vi "Report Tool2.vi"(0 "name or relative path":string=".csv", 1 "Files":path[](array[path]), 5 "base path":path=path "C:/RageATE Results", 13 "WriteToFile(t)":bool=TRUE) -> (4 "reportfile(str)":string="C:\\RageATE Results\\1234.csv.csv")   [LabVIEW 2018]
uses:
  <vilib>/Utility/file.llb/Read Delimited Spreadsheet (string).vi
  <vilib>/Utility/file.llb/Write Delimited Spreadsheet (string).vi
panel:
  out "file or folder exists?":bool
  out "reportfile":path=path "C:/RageATE Results/1234.csv.csv"
  out "Tx-Att_Test Name":string
  out "Tx_Test Name":string
  in  "RunRx(t)":bool=TRUE
  in  "RunTx(t)":bool=TRUE
  in  "RunATTEN(t)":bool=TRUE
  in  "error in (no error)":errorcluster
  out "error out":errorcluster
  out "TX-ATT_DAT":string[][](array[string])=[["#Test Name:", "REV-C_TETRA_TX-ATTEN"], ["#MSN:", "RGE2100000"], ["#ESN:", "xxxxxxxx"], ["#TestOperator:", "411 WATSON T NBPT"], ["#Test_Bench_Name:", "WAM_PROD_TEST-1"], ["#Test Parameters File Name:", "'C:\\RageATE\\Automated Tests\\Tetra WAM\\PRODUCTION\\setup files\\WAM-C_TX-ATTEN_Parameters.tst'"], ["#Gitlog Commit:", "41159ffc8fe9c2318ec8f6db4e89b94d30bdf9e8"], ["#LotID:", "2228"], ["#SW_Version:", "02000005"], ["#Result File Path:", "'C:\\RageATE Results\\REV-C_TETRA_TX-ATTEN\\7_11_2022\\REV-C_TETRA_TX-ATTEN_SN_RGE2100000_ 2228_071122-130320.csv'"], ["%TX_ATT", "PASS"]]
  out "TX_ATT":string="PASS"
  out "TxAtt_DataLength":i32=24
  out "TxAtt_Result":i32[][](array[numeric])=[[1], [1], [1], [1], [1], [1], [1], [1], [1], [1], [1], [1], [1], [1], [1], [1], [1], [1], [1], [1], [1], [1], [1], [1]]
  out "TxAtt_DataHeaderRow":i32=45
  out "TxAtt_Header_data":string[](array[string])=["REV-C_TETRA_TX-ATTEN", "RGE2100000", "xxxxxxxx", "411 WATSON T NBPT", "WAM_PROD_TEST-1", "'C:\\RageATE\\Automated Tests\\Tetra WAM\\PRODUCTION\\setup files\\WAM-C_TX-ATTEN_Parameters.tst'", "41159ffc8fe9c2318ec8f6db4e89b94d30bdf9e8", "2228", "02000005", "'C:\\RageATE Results\\REV-C_TETRA_TX-ATTEN\\7_11_2022\\REV-C_TETRA_TX-ATTEN_SN_RGE2100000_ 2228_071122-130320.csv'"]
  out "TxAtt_Header":string[](array[string])=["#Test Name:", "#MSN:", "#ESN:", "#TestOperator:", "#Test_Bench_Name:", "#Test Parameters File Name:", "#Gitlog Commit:", "#LotID:", "#SW_Version:", "#Result File Path:"]
  out "TXAtt_ResultFile":string="C:\\RageATE Results\\REV-C_TETRA_TX-ATTEN\\7_11_2022\\REV-C_TETRA_TX-ATTEN_SN_RGE2100000_ 2228_071122-130320.csv"
  in  "TX_PROD_ATTEN":path=path "C:/RageATE Results/REV-C_TETRA_TX-ATTEN/7_11_2022/REV-C_TETRA_TX-ATTEN_SN_RGE2100000_ 2228_071122-130320.csv"
  out "TxAtt_Data":string[][](array[string])
  out "TX_FLAT":string="FAIL *12"
  out "RX_DAT":string[][](array[string])=[["#Test Name:", "REV-C_TETRA_RX-PROD"], ["#MSN:", "RGE2100000"], ["#ESN:", "xxxxxxxx"], ["#TestOperator:", "411 WATSON T NBPT"], ["#Test_Bench_Name:", "WAM_PROD_TEST-1"], ["#Test Parameters File Name:", "'C:\\RageATE\\Automated Tests\\Tetra WAM\\PRODUCTION\\setup files\\WAM-C_RX-PROD_Parameters.tst'"], ["#Gitlog Commit:", "41159ffc8fe9c2318ec8f6db4e89b94d30bdf9e8"], ["#LotID:", "2228"], ["#SW_Version: ", "02000005"], ["#Result File Path:", "'C:\\RageATE Results\\REV-C_TETRA_RX-PROD\\7_11_2022\\REV-C_TETRA_RX-PROD_SN_RGE2100000_ 2228_071122-132555.csv'"], ["%RX_DC", "PASS"], ["%RX_GAIN", "PASS"], ["%RX_NF", "FAIL *34"]]
  out "RX_DC":string="PASS"
  out "RX_G":string="PASS"
  out "RX_NF":string="FAIL *34"
  out "Rx_DataLength":i32=1608
  out "Rx_Result":i32[][](array[numeric])
  out "Rx_DataHeaderRow":i32=45
  out "Rx_Header_data":string[](array[string])=["REV-C_TETRA_RX-PROD", "RGE2100000", "xxxxxxxx", "411 WATSON T NBPT", "WAM_PROD_TEST-1", "'C:\\RageATE\\Automated Tests\\Tetra WAM\\PRODUCTION\\setup files\\WAM-C_RX-PROD_Parameters.tst'", "41159ffc8fe9c2318ec8f6db4e89b94d30bdf9e8", "2228", "02000005", "'C:\\RageATE Results\\REV-C_TETRA_RX-PROD\\7_11_2022\\REV-C_TETRA_RX-PROD_SN_RGE2100000_ 2228_071122-132555.csv'"]
  out "Rx_Header":string[](array[string])=["#Test Name:", "#MSN:", "#ESN:", "#TestOperator:", "#Test_Bench_Name:", "#Test Parameters File Name:", "#Gitlog Commit:", "#LotID:", "#SW_Version: ", "#Result File Path:"]
  out "RX_ResultFile":string="C:\\RageATE Results\\REV-C_TETRA_RX-PROD\\7_11_2022\\REV-C_TETRA_RX-PROD_SN_RGE2100000_ 2228_071122-132555.csv"
  in  "RX_PROD_FILE":path=path "C:/RageATE Results/REV-C_TETRA_RX-PROD/7_11_2022/REV-C_TETRA_RX-PROD_SN_RGE2100000_ 2228_071122-132555.csv"
  out "Rx_Data":string[][](array[string])
  out "Tx_Result":i32[][](array[numeric])
  out "Tx_DataLength":i32=2412
  out "Tx_Header":string[](array[string])=["#Test Name:", "#ESN:", "#MSN:", "#TestOperator:", "#Test_Bench_Name:", "#Test Parameters File Name:", "#Gitlog Commit:", "#LotID:", "#SW_Version: ", "#Result File Path:"]
  out "Tx_Data":string[][](array[string])
  out "TX_DAT":string[][](array[string])=[["#Test Name:", "REV-C_TETRA_TX-PROD"], ["#ESN:", "xxxxxxxx"], ["#MSN:", "RGE2100000"], ["#TestOperator:", "411 WATSON T NBPT"], ["#Test_Bench_Name:", "WAM_PROD_TEST-1"], ["#Test Parameters File Name:", "'C:\\RageATE\\Automated Tests\\Tetra WAM\\PRODUCTION\\setup files\\WAM-C_TX-PROD_Parameters.tst'"], ["#Gitlog Commit:", "41159ffc8fe9c2318ec8f6db4e89b94d30bdf9e8"], ["#LotID:", "2228"], ["#SW_Version: ", "02000005"], ["#Result File Path:", "'C:\\RageATE Results\\REV-C_TETRA_TX-PROD\\7_11_2022\\REV-C_TETRA_TX-PROD_SN_RGE2100000_ 2228_071122-130423.csv'"], ["%TX_DC", "PASS"], ["%TX_POW", "FAIL *1301"], ["%TX_S11", "FAIL *125"], ["%TX_H2", "PASS"], ["%TX_FLAT", "FAIL *12"]]
  out "Tx_Header_data":string[](array[string])=["REV-C_TETRA_TX-PROD", "xxxxxxxx", "RGE2100000", "411 WATSON T NBPT", "WAM_PROD_TEST-1", "'C:\\RageATE\\Automated Tests\\Tetra WAM\\PRODUCTION\\setup files\\WAM-C_TX-PROD_Parameters.tst'", "41159ffc8fe9c2318ec8f6db4e89b94d30bdf9e8", "2228", "02000005", "'C:\\RageATE Results\\REV-C_TETRA_TX-PROD\\7_11_2022\\REV-C_TETRA_TX-PROD_SN_RGE2100000_ 2228_071122-130423.csv'"]
  in  "TX_PROD_FILE":path=path "C:/RageATE Results/REV-C_TETRA_TX-PROD/7_11_2022/REV-C_TETRA_TX-PROD_SN_RGE2100000_ 2228_071122-130423.csv"
  out "TX_ResultFile":string="C:\\RageATE Results\\REV-C_TETRA_TX-PROD\\7_11_2022\\REV-C_TETRA_TX-PROD_SN_RGE2100000_ 2228_071122-130423.csv"
  out "Tx_DataHeaderRow":i32=45
  out "Rx_Test Name":string
  out "TX_H2":string="PASS"
  out "TX_S11":string="FAIL *125"
  out "TX_POW":string="FAIL *1301"
  out "TX_DC":string="PASS"
  # "C:\\RageATE Results\\REV-C_TETRA_TX-ATTEN\\7_11_2022\\REV-C_TETRA_TX-ATTEN_SN_RGE2100000_ 2228_071122-130320.csv"
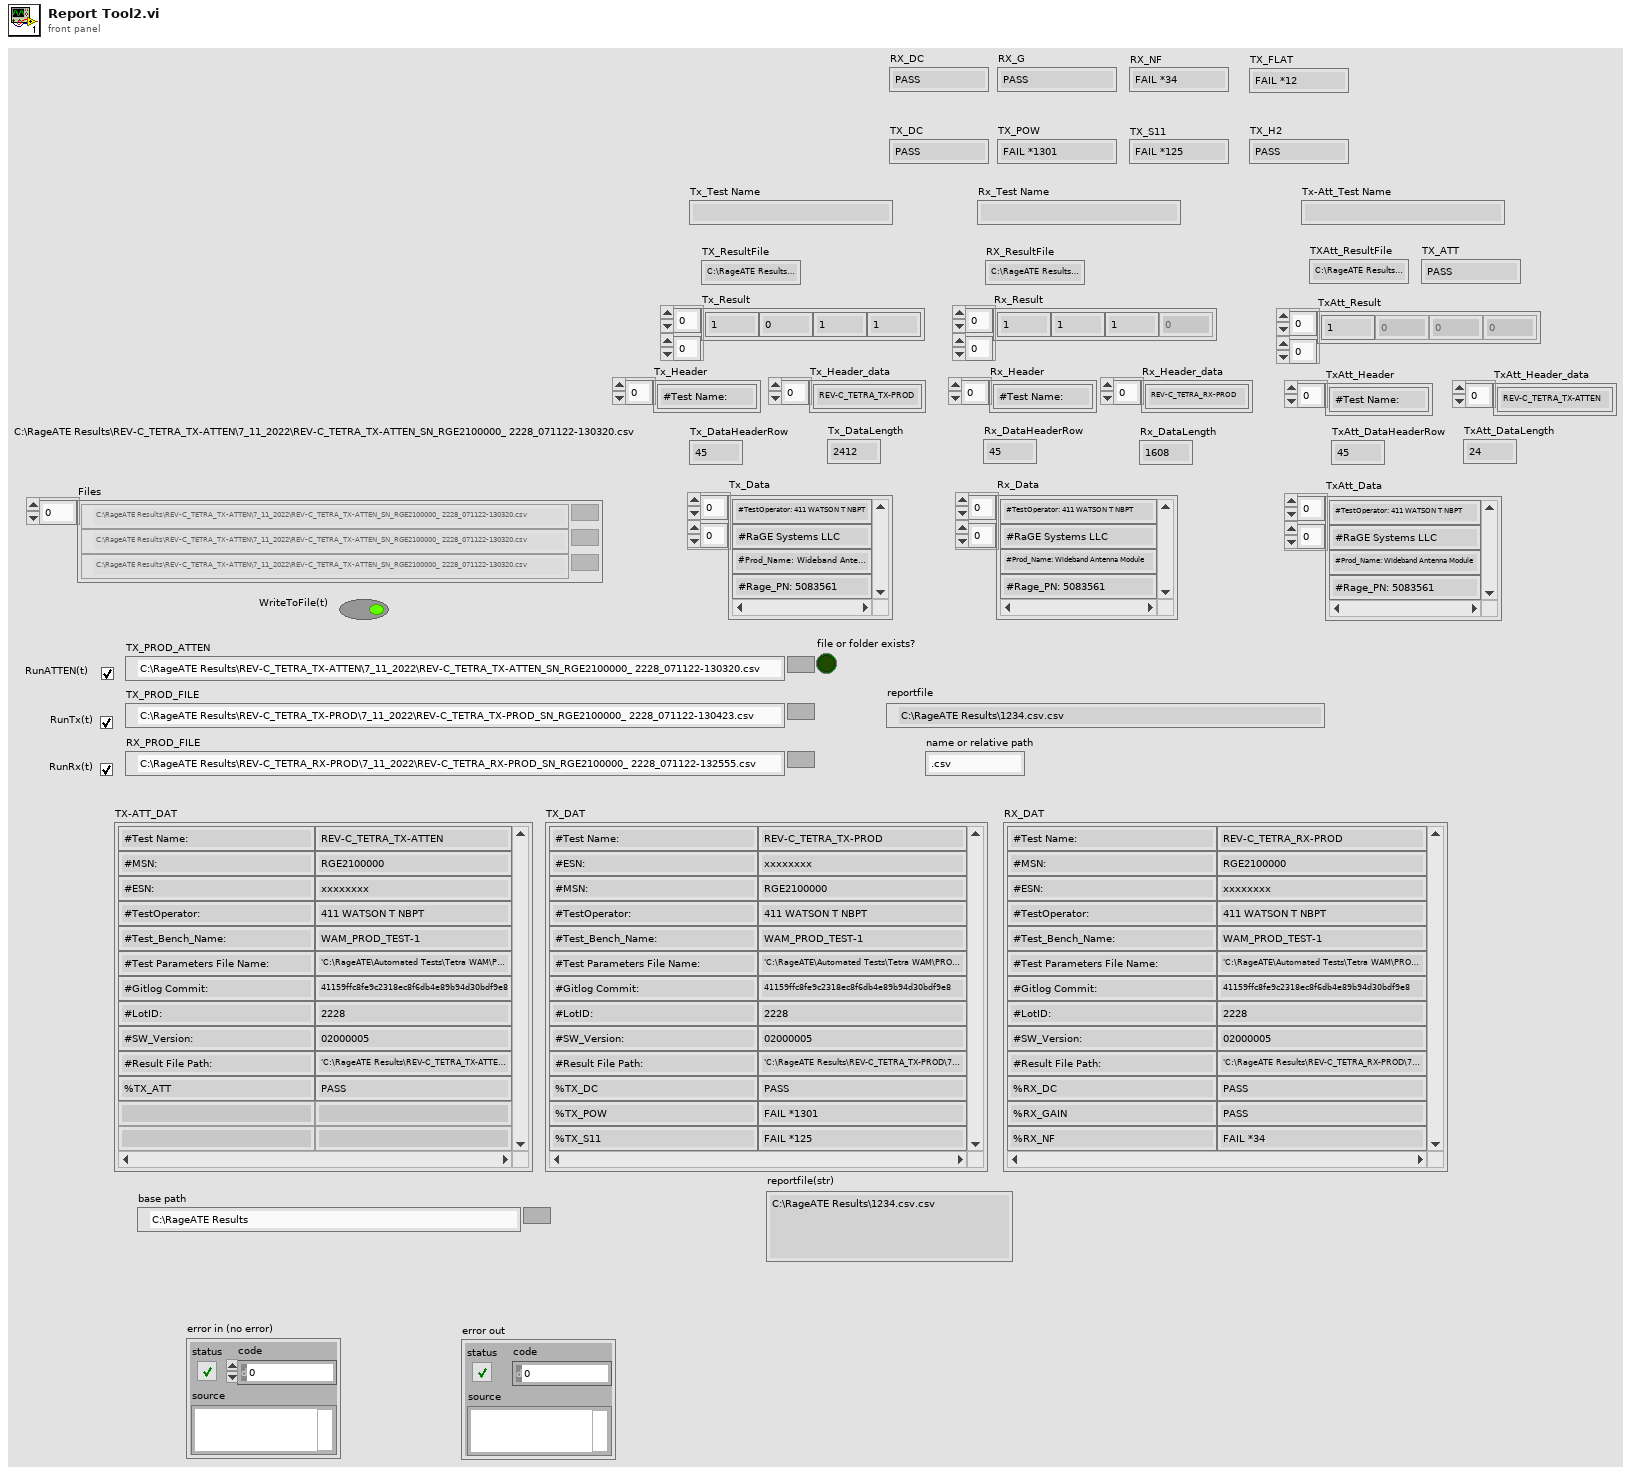
[diagram p1: front panel]
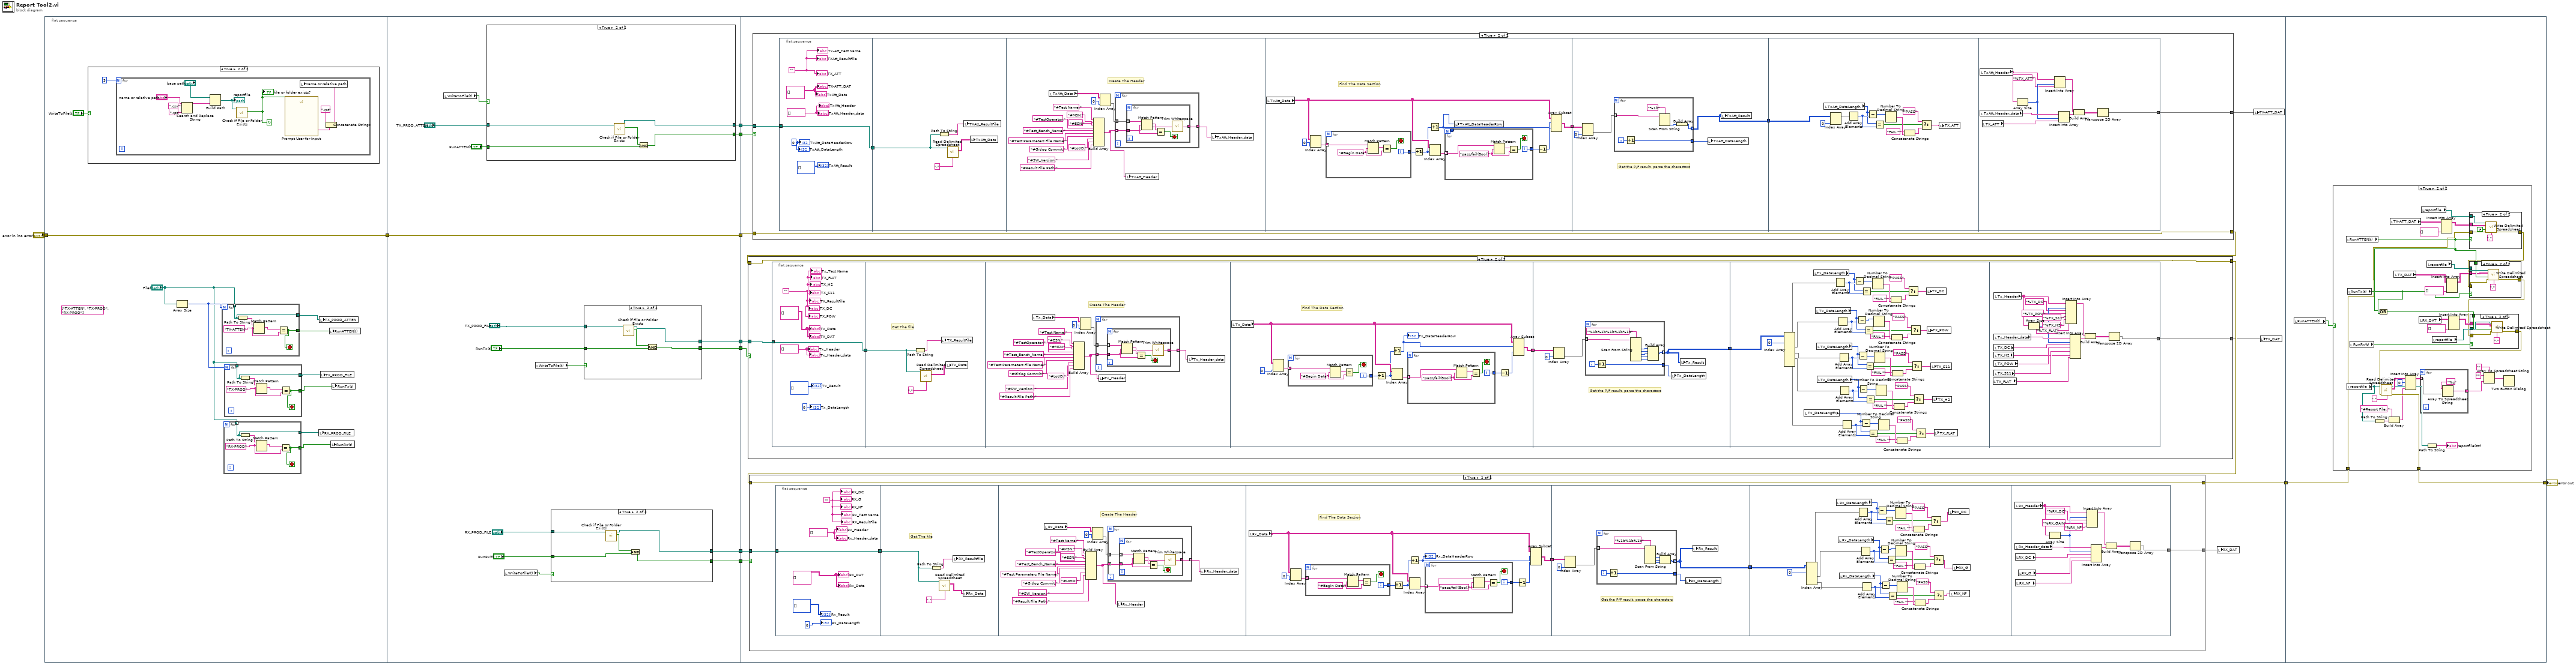
[diagram p0: block diagram]
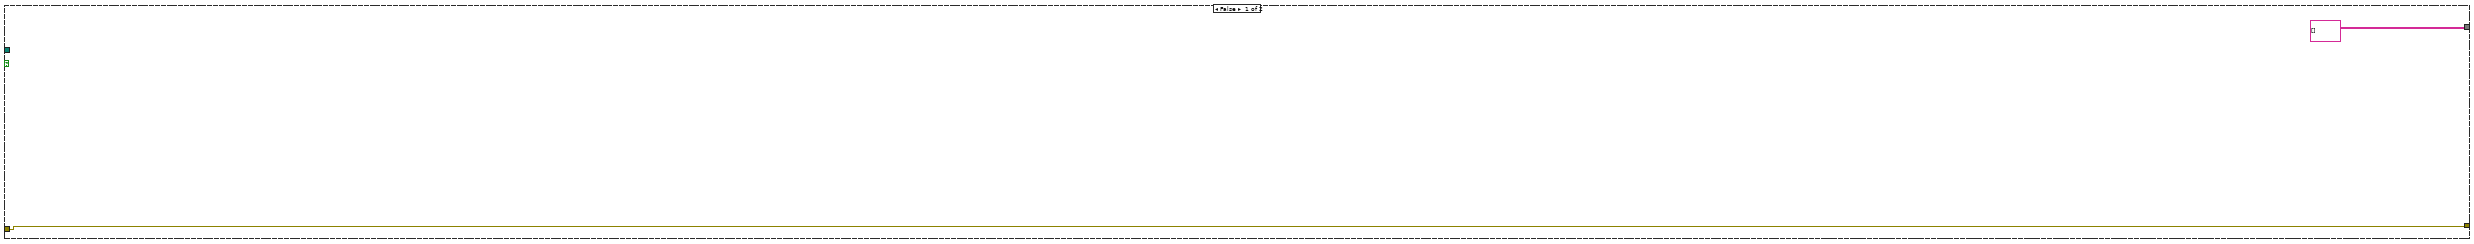
[diagram p6: hidden frame]
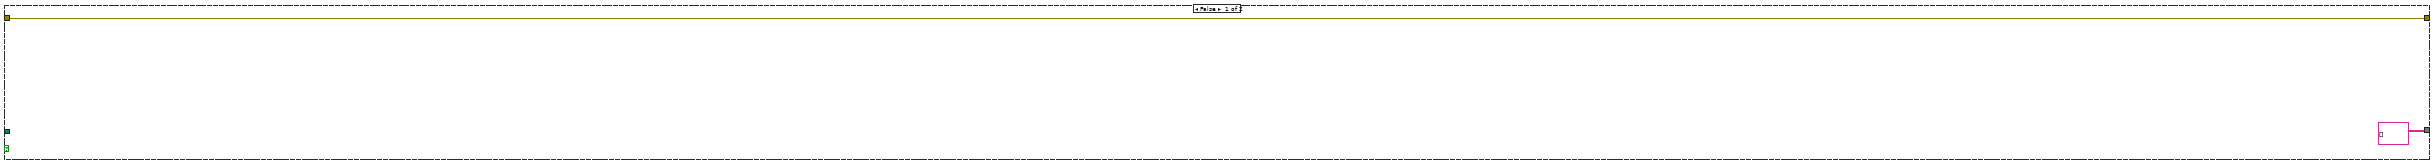
[diagram p7: hidden frame]
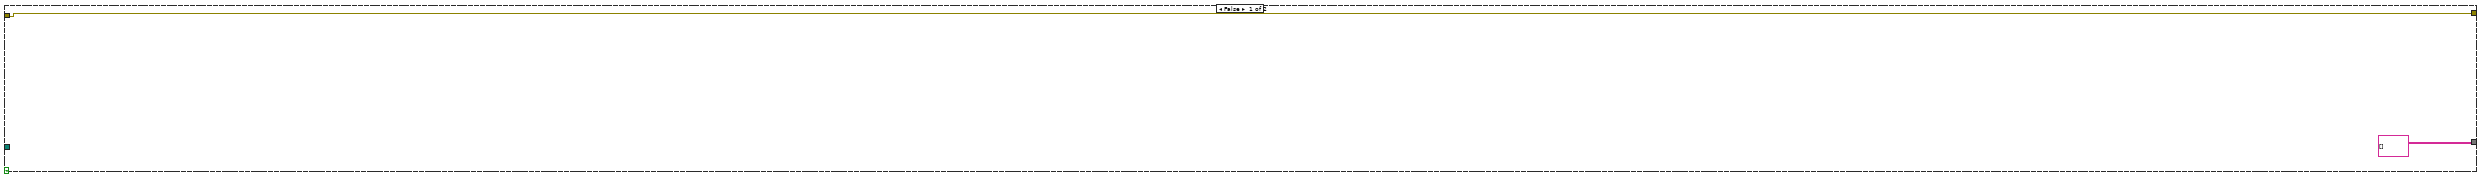
[diagram p8: hidden frame]
diagram:
  n1 = flat-sequence {
    tunnel: "error in (no error)" -> [w21]
    tunnel: [w21] -> w1
    tunnel: [w61] -> w8
    tunnel: [w62] -> w7
    tunnel: [w57] -> w6
    tunnel: [w58] -> w5
    tunnel: [w53] -> w4
    tunnel: [w54] -> w3
    tunnel: [w63] -> w2
    tunnel: w1 -> [w63]
    tunnel: [w88] -> w9
    tunnel: w8 -> [w97]
    tunnel: w7 -> [w96]
    tunnel: w6 -> [w95]
    tunnel: w5 -> [w94]
    tunnel: w4 -> [w93]
    tunnel: w3 -> [w92]
    tunnel: w2 -> [w91]
    tunnel: [w460] -> w10
    tunnel: w9 -> [w461]
    frame #0 {
      (unwired) string[] ["TX-ATTEN", "TX-PROD", "RX-PROD"] ("string")
      n2 = case shown="True" "WriteToFile(t)" {
        frame False {
        }
        frame True {
          n3 = for {
            N: 3 -> [_]
            stop <- w45 continue-if-true
            n4 = Search and Replace String(input string="name or relative path", search string=".csv", replace string=".rpt" ("replace string (\"\")")) -> (result string=w41:string)  [unwired: 5 in, 3 out]
            n5 = Build Path(base path="base path", name or relative path=w41) -> (appended path=w46:path)
            "reportfile" <- w46
            n6 = call <vilib>:"Check if File or Folder Exists.vi"("path"=w46) -> ("file or folder exists?"=w45:bool)  [unwired: 8 in, 2 out]
            "file or folder exists?" <- w45
            n7 = call "Prompt User for Input"("Enable"=w45) -> ("Filename"=w44:string)  [unwired: 16 in, 2 out]
            n8 = Concatenate Strings(w44, ".rpt" ("string")) -> (w43:string)
            n9 = local write "name or relative path"(w43) -> ()
          }
        }
      }
      n10 = Array Size(array="Files") -> (size(s)=w17:i32)
      n11 = for {
        N: w17 -> [_]
        tunnel: "Files" -> [w33] mode=indexing
        tunnel: [w32] -> w19
        tunnel: [w33] -> w18
        stop <- w32 stop-if-true
        w34 = "TX-ATTEN" ("string")
        n12 = Path To String(path=w33) -> (string=w36:string)
        n13 = Match Pattern(string=w36, regular expression=w34) -> (match substring=w35:string)  [unwired: 1 in, 3 out]
        n14 = Equal?(x=w35, y=w34) -> (x = y?=w32:bool)
      }
      n15 = for {
        tunnel: "Files" -> [w23] mode=indexing
        tunnel: [w22] -> w12
        tunnel: [w23] -> w13
        stop <- w22 stop-if-true
        w24 = "RX-PROD" ("string")
        n16 = Path To String(path=w23) -> (string=w26:string)
        n17 = Match Pattern(string=w26, regular expression=w24) -> (match substring=w25:string)  [unwired: 1 in, 3 out]
        n18 = Equal?(x=w25, y=w24) -> (x = y?=w22:bool)
      }
      n19 = for {
        N: w17 -> [_]
        tunnel: "Files" -> [w28] mode=indexing
        tunnel: [w27] -> w15
        tunnel: [w28] -> w16
        stop <- w27 stop-if-true
        w29 = "TX-PROD" ("string")
        n20 = Path To String(path=w28) -> (string=w31:string)
        n21 = Match Pattern(string=w31, regular expression=w29) -> (match substring=w30:string)  [unwired: 1 in, 3 out]
        n22 = Equal?(x=w30, y=w29) -> (x = y?=w27:bool)
      }
      n23 = local write "RX_PROD_FILE"(w13) -> ()
      n24 = local write "TX_PROD_ATTEN"(w18) -> ()
      n25 = local write "TX_PROD_FILE"(w16) -> ()
      n26 = local write "RunATTEN(t)"(w19) -> ()
      n27 = local write "RunRx(t)"(w12) -> ()
      n28 = local write "RunTx(t)"(w15) -> ()
    }
    frame #1 {
      n29 = local read "WriteToFile(t)"() -> (w52:bool)
      n30 = case shown="True" w52 {
        tunnel: [w78 w83] -> w62
        tunnel: [w79 w82] -> w61
        tunnel: "TX_PROD_ATTEN" -> [w79 w81]
        tunnel: "RunATTEN(t)" -> [w78 w80]
        frame False {
        }
        frame True {
          n31 = call <vilib>:"Check if File or Folder Exists.vi"("path"=w81) -> ("file or folder exists?"=w84:bool, "dup path"=w82:path)  [unwired: 8 in, 1 out]
          n32 = And(x=w84, y=w80) -> (x .and. y?=w83:bool)
        }
      }
      n33 = local read "WriteToFile(t)"() -> (w49:bool)
      n34 = local read "WriteToFile(t)"() -> (w50:bool)
      n35 = case shown="True" w49 {
        tunnel: "RX_PROD_FILE" -> [w64 w70]
        tunnel: "RunRx(t)" -> [w65 w69]
        tunnel: [w65 w67] -> w54
        tunnel: [w64 w66] -> w53
        frame False {
        }
        frame True {
          n36 = call <vilib>:"Check if File or Folder Exists.vi"("path"=w70) -> ("file or folder exists?"=w68:bool, "dup path"=w66:path)  [unwired: 8 in, 1 out]
          n37 = And(x=w68, y=w69) -> (x .and. y?=w67:bool)
        }
      }
      n38 = case shown="True" w50 {
        tunnel: "RunTx(t)" -> [w72 w77]
        tunnel: "TX_PROD_FILE" -> [w71 w75]
        tunnel: [w72 w74] -> w58
        tunnel: [w71 w73] -> w57
        frame False {
        }
        frame True {
          n39 = call <vilib>:"Check if File or Folder Exists.vi"("path"=w75) -> ("file or folder exists?"=w76:bool, "dup path"=w73:path)  [unwired: 8 in, 1 out]
          n40 = And(x=w76, y=w77) -> (x .and. y?=w74:bool)
        }
      }
    }
    frame #2 {
      n41 = case shown="True" w96 {
        tunnel: w97 -> [_ w102]
        tunnel: [string[][] [] w101] -> w85
        tunnel: w91 -> [w98 w100]
        tunnel: [w98 w100] -> w90
        frame False {
        }
        frame True {
          n42 = flat-sequence {
            tunnel: [w107] -> w103
            tunnel: w102 -> [w107]
            tunnel: w103 -> [w112]
            tunnel: [w141] -> w105
            tunnel: w105 -> [w164]
            tunnel: [w161] -> w104
            tunnel: w104 -> [w172]
            tunnel: [w184] -> w101
            frame #0 {
              w106 = ""
              w111 = 0 ("TxAtt_DataHeaderRow")
              w108 = string[] [] ("TxAtt_Header_data")
              w109 = string[][] [] ("TX_DAT")
              "TXAtt_ResultFile" <- w106
              "TxAtt_Data" <- w109
              "TxAtt_Header" <- w108
              "TxAtt_Header_data" <- w108
              "TxAtt_DataHeaderRow" <- w111
              "TxAtt_Result" <- i32[][] [] ("TxAtt_Result")
              "TxAtt_DataLength" <- w111
              "TX_ATT" <- w106
              "TX-ATT_DAT" <- w109
              "Tx-Att_Test Name" <- w106
            }
            frame #1 {
              n43 = Path To String(path=w112) -> (string=w114:string)
              n44 = call-poly <vilib>:"Read Delimited Spreadsheet.vi"("file path (dialog if empty)"=w112, "delimiter (\\t)"="," ("delimiter (\\t)")) -> ("all rows"=w113:string[][])  [unwired: 8 in, 5 out]
              n45 = local write "TXAtt_ResultFile"(w114) -> ()
              n46 = local write "TxAtt_Data"(w113) -> ()
            }
            frame #2 {
              # "Create The Header"
              n47 = local read "TxAtt_Data"() -> (w122:string[][])
              n48 = Build Array("#Test Name:" ("regular expression"), "#MSN:" ("regular expression"), "#ESN:" ("regular expression"), "#TestOperator:" ("regular expression"), "#Test_Bench_Name:" ("regular expression"), "#Test Parameters File Name:" ("regular expression"), "#Gitlog Commit:" ("regular expression"), "#LotID:" ("regular expression"), "#SW_Version:" ("regular expression"), "#Result File Path:" ("regular expression")) -> (w121:string[])
              n49 = Index Array(array=w122, index (col)=0 ("disabled index (col)")) -> (element=w130:string[])  [unwired: 1 in]
              n50 = for {
                tunnel: w121 -> [w133] mode=indexing
                tunnel: w130 -> [w132]
                tunnel: [w131] -> w120 mode=indexing
                n51 = for {
                  tunnel: w133 -> [w134]
                  tunnel: [w136] -> w131
                  tunnel: w132 -> [w135] mode=indexing
                  stop <- w139 stop-if-true
                  n52 = Match Pattern(string=w135, regular expression=w134) -> (match substring=w138:string, after substring=w137:string)  [unwired: 1 in, 2 out]
                  n53 = Equal?(x=w138, y=w134) -> (x = y?=w139:bool)
                  n54 = call <vilib>:"Trim Whitespace.vi"("string"=w137) -> ("trimmed string"=w136:string)  [unwired: 1 in]
                }
              }
              n55 = local write "TxAtt_Header"(w121) -> ()
              n56 = local write "TxAtt_Header_data"(w120) -> ()
            }
            frame #3 {
              # "Find The Data Section"
              n57 = local read "TxAtt_Data"() -> (w149:string[][])
              n58 = Index Array(array=w149, index (col)=0 ("disabled index (col)")) -> (element=w143:string[])  [unwired: 1 in]
              n59 = for {
                tunnel: w143 -> [w160] mode=indexing
                tunnel: [w156] -> w144
                i -> [w156]
                stop <- w157 stop-if-true
                w158 = "#Begin Data" ("regular expression")
                n60 = Match Pattern(string=w160, regular expression=w158) -> (match substring=w159:string)  [unwired: 1 in, 3 out]
                n61 = Equal?(x=w159, y=w158) -> (x = y?=w157:bool)
              }
              n62 = Increment(x=w144) -> (x+1=w146:i32)
              n63 = Increment(x=w146) -> (x+1=w140:i32)
              n64 = Index Array(array=w149, index (row)=w146) -> (element=w145:string[])  [unwired: 1 in]
              n65 = for {
                N -> [w150]
                tunnel: w145 -> [w155] mode=indexing
                tunnel: [w151] -> w147
                tunnel: [w150] -> _
                i -> [w151]
                stop <- w152 stop-if-true
                w153 = "pass/fail(Bool)" ("regular expression")
                n66 = Match Pattern(string=w155, regular expression=w153) -> (match substring=w154:string)  [unwired: 1 in, 3 out]
                n67 = Equal?(x=w154, y=w153) -> (x = y?=w152:bool)
              }
              n68 = local write "TxAtt_DataHeaderRow"(w140) -> ()
              n69 = Decrement(x=w147) -> (x-1=w148:i32)
              n70 = Array Subset(array=w149, index (row)=w140, index (col)=w148) -> (w141:string[][])  [unwired: 2 in]
            }
            frame #4 {
              # "Get the P/F result, parse the charactors"
              n71 = Index Array(array=w164, index (col)=0 ("disabled index (col)")) -> (element=w165:string[])  [unwired: 1 in]
              n72 = for {
                tunnel: w165 -> [w170] mode=indexing
                tunnel: [w169] -> w161 mode=indexing
                tunnel: [w166] -> w162
                i -> [w167]
                n73 = Increment(x=w167) -> (x+1=w166:i32)
                n74 = Scan From String(format string="%1b", input string=w170) -> (output 1=w168:i32)  [unwired: 3 in, 3 out]
                n75 = Build Array(w168) -> (w169:i32[])
              }
              n76 = local write "TxAtt_DataLength"(w162) -> ()
              n77 = local write "TxAtt_Result"(w161) -> ()
            }
            frame #5 {
              n78 = local read "TxAtt_DataLength"() -> (w176:i32)
              n79 = Index Array(array=w172, index (col)=0 ("disabled index (col)")) -> (element=w179:i32[])  [unwired: 1 in]
              n80 = Add Array Elements(numeric array=w179) -> (sum=w177:i32)
              n81 = Subtract(x=w176, y=w177) -> (x-y=w180:i32)
              n82 = Equal?(x=w176, y=w177) -> (x = y?=w178:bool)
              n83 = Number To Decimal String(number=w180) -> (decimal integer string=w182:string)  [unwired: 1 in]
              n84 = Concatenate Strings("FAIL *" ("f"), w182) -> (w181:string)
              n85 = Select(t="PASS", s=w178, f=w181) -> (s? t:f=w183:string)
              n86 = local write "TX_ATT"(w183) -> ()
            }
            frame #6 {
              n87 = local read "TxAtt_Header"() -> (w191:string[])
              n88 = local read "TxAtt_Header_data"() -> (w192:string[])
              n89 = local read "TX_ATT"() -> (w185:string)
              n90 = Array Size(array=w191) -> (size(s)=w190:i32)
              n91 = Insert Into Array(array=w191, index=w190, new element="%TX_ATT" ("new element/subarray")) -> (w188:string[])
              n92 = Insert Into Array(array=w192, index=w190, new element=w185) -> (w189:string[])
              n93 = Build Array(w188, w189) -> (w187:string[][])
              n94 = Transpose 2D Array(2D array=w187) -> (transposed array=w184:string[][])
            }
          }
        }
      }
      n95 = case shown="True" w94 {
        tunnel: w95 -> [_ w317]
        tunnel: [string[][] [] w316] -> w86
        tunnel: w90 -> [w313 w315]
        tunnel: [w313 w315] -> w89
        frame False {
        }
        frame True {
          n96 = flat-sequence {
            tunnel: [w322] -> w318
            tunnel: w317 -> [w322]
            tunnel: w318 -> [w327]
            tunnel: [w355] -> w320
            tunnel: w320 -> [w378]
            tunnel: [w375] -> w319
            tunnel: w319 -> [w396]
            tunnel: [w442] -> w316
            frame #0 {
              w321 = ""
              w326 = string[] [] ("TxAtt_Header_data")
              w325 = string[][] [] ("TX_DAT")
              "Tx_Header_data" <- w326
              "Tx_Header" <- w326
              "Tx_DataLength" <- 0 ("Tx_DataLength")
              "Tx_Result" <- i32[][] [] ("Tx_Result")
              "TX_DC" <- w321
              "TX_POW" <- w321
              "TX_S11" <- w321
              "TX_H2" <- w321
              "TX_FLAT" <- w321
              "TX_DAT" <- w325
              "TX_ResultFile" <- w321
              "Tx_Data" <- w325
              "Tx_Test Name" <- w321
            }
            frame #1 {
              # "Get The file"
              n97 = Path To String(path=w327) -> (string=w329:string)
              n98 = call-poly <vilib>:"Read Delimited Spreadsheet.vi"("file path (dialog if empty)"=w327, "delimiter (\\t)"="," ("delimiter (\\t)")) -> ("all rows"=w328:string[][])  [unwired: 8 in, 5 out]
              n99 = local write "TX_ResultFile"(w329) -> ()
              n100 = local write "Tx_Data"(w328) -> ()
            }
            frame #2 {
              # "Create The Header"
              n101 = local read "Tx_Data"() -> (w337:string[][])
              n102 = Build Array("#Test Name:" ("regular expression"), "#ESN:" ("regular expression"), "#MSN:" ("regular expression"), "#TestOperator:" ("regular expression"), "#Test_Bench_Name:" ("regular expression"), "#Test Parameters File Name:" ("regular expression"), "#Gitlog Commit:" ("regular expression"), "#LotID:" ("regular expression"), "#SW_Version: " ("regular expression"), "#Result File Path:" ("regular expression")) -> (w335:string[])
              n103 = Index Array(array=w337, index (col)=0 ("disabled index (col)")) -> (element=w345:string[])  [unwired: 1 in]
              n104 = for {
                tunnel: w335 -> [w348] mode=indexing
                tunnel: w345 -> [w347]
                tunnel: [w346] -> w336 mode=indexing
                n105 = for {
                  tunnel: w348 -> [w349]
                  tunnel: [w351] -> w346
                  tunnel: w347 -> [w350] mode=indexing
                  stop <- w354 stop-if-true
                  n106 = Match Pattern(string=w350, regular expression=w349) -> (match substring=w353:string, after substring=w352:string)  [unwired: 1 in, 2 out]
                  n107 = Equal?(x=w353, y=w349) -> (x = y?=w354:bool)
                  n108 = call <vilib>:"Trim Whitespace.vi"("string"=w352) -> ("trimmed string"=w351:string)  [unwired: 1 in]
                }
              }
              n109 = local write "Tx_Header"(w335) -> ()
              n110 = local write "Tx_Header_data"(w336) -> ()
            }
            frame #3 {
              # "Find The Data Section"
              n111 = local read "Tx_Data"() -> (w364:string[][])
              n112 = Index Array(array=w364, index (col)=0 ("disabled index (col)")) -> (element=w357:string[])  [unwired: 1 in]
              n113 = for {
                tunnel: w357 -> [w374] mode=indexing
                tunnel: [w370] -> w358
                i -> [w370]
                stop <- w371 stop-if-true
                w372 = "#Begin Data" ("regular expression")
                n114 = Match Pattern(string=w374, regular expression=w372) -> (match substring=w373:string)  [unwired: 1 in, 3 out]
                n115 = Equal?(x=w373, y=w372) -> (x = y?=w371:bool)
              }
              n116 = Increment(x=w358) -> (x+1=w360:i32)
              n117 = Increment(x=w360) -> (x+1=w363:i32)
              "Tx_DataHeaderRow" <- w363
              n118 = Index Array(array=w364, index (row)=w360) -> (element=w359:string[])  [unwired: 1 in]
              n119 = for {
                tunnel: w359 -> [w369] mode=indexing
                tunnel: [w365] -> w361
                i -> [w365]
                stop <- w366 stop-if-true
                w367 = "pass/fail(Bool)" ("regular expression")
                n120 = Match Pattern(string=w369, regular expression=w367) -> (match substring=w368:string)  [unwired: 1 in, 3 out]
                n121 = Equal?(x=w368, y=w367) -> (x = y?=w366:bool)
              }
              n122 = Decrement(x=w361) -> (x-1=w362:i32)
              n123 = Array Subset(array=w364, index (row)=w363, index (col)=w362) -> (w355:string[][])  [unwired: 2 in]
            }
            frame #4 {
              # "Get the P/F result, parse the charactors"
              n124 = Index Array(array=w378, index (col)=0 ("disabled index (col)")) -> (element=w379:string[])  [unwired: 1 in]
              n125 = for {
                tunnel: w379 -> [w388] mode=indexing
                tunnel: [w384] -> w375 mode=indexing
                tunnel: [w381] -> w376
                i -> [w382]
                n126 = Increment(x=w382) -> (x+1=w381:i32)
                n127 = Scan From String(format string="%1b%1b%1b%1b%1b", input string=w388) -> (output 1=w383:i32, output 2=w387:i32, output 3=w386:i32, output 4=w385:i32, output 5=w380:i32)  [unwired: 7 in, 3 out]
                n128 = Build Array(w383, w387, w386, w385, w380) -> (w384:i32[])
              }
              n129 = local write "Tx_DataLength"(w376) -> ()
              n130 = local write "Tx_Result"(w375) -> ()
            }
            frame #5 {
              n131 = Index Array(array=w396, index (col) #1=0 ("disabled index (col)")) -> (element #1=w421:i32[], element #2=w420:i32[], element #3=w419:i32[], element #4=w418:i32[], element #5=w441:i32[])  [unwired: 9 in]
              n132 = local read "Tx_DataLength"() -> (w439:i32)
              n133 = local read "Tx_DataLength"() -> (w415:i32)
              n134 = local read "Tx_DataLength"() -> (w414:i32)
              n135 = local read "Tx_DataLength"() -> (w409:i32)
              n136 = local read "Tx_DataLength"() -> (w408:i32)
              n137 = Add Array Elements(numeric array=w421) -> (sum=w416:i32)
              n138 = Add Array Elements(numeric array=w420) -> (sum=w413:i32)
              n139 = Add Array Elements(numeric array=w419) -> (sum=w410:i32)
              n140 = Add Array Elements(numeric array=w418) -> (sum=w407:i32)
              n141 = Add Array Elements(numeric array=w441) -> (sum=w440:i32)
              n142 = Subtract(x=w415, y=w416) -> (x-y=w422:i32)
              n143 = Subtract(x=w414, y=w413) -> (x-y=w425:i32)
              n144 = Subtract(x=w409, y=w410) -> (x-y=w428:i32)
              n145 = Subtract(x=w408, y=w407) -> (x-y=w433:i32)
              n146 = Subtract(x=w439, y=w440) -> (x-y=w436:i32)
              n147 = Equal?(x=w415, y=w416) -> (x = y?=w417:bool)
              n148 = Equal?(x=w414, y=w413) -> (x = y?=w412:bool)
              n149 = Equal?(x=w409, y=w410) -> (x = y?=w411:bool)
              n150 = Equal?(x=w408, y=w407) -> (x = y?=w434:bool)
              n151 = Equal?(x=w439, y=w440) -> (x = y?=w435:bool)
              n152 = Number To Decimal String(number=w422) -> (decimal integer string=w424:string)  [unwired: 1 in]
              n153 = Number To Decimal String(number=w425) -> (decimal integer string=w427:string)  [unwired: 1 in]
              n154 = Number To Decimal String(number=w428) -> (decimal integer string=w430:string)  [unwired: 1 in]
              n155 = Number To Decimal String(number=w433) -> (decimal integer string=w431:string)  [unwired: 1 in]
              n156 = Number To Decimal String(number=w436) -> (decimal integer string=w438:string)  [unwired: 1 in]
              n157 = Concatenate Strings("FAIL *" ("f"), w424) -> (w423:string)
              n158 = Concatenate Strings("FAIL *" ("f"), w427) -> (w426:string)
              n159 = Concatenate Strings("FAIL *" ("f"), w430) -> (w429:string)
              n160 = Concatenate Strings("FAIL *" ("f"), w431) -> (w432:string)
              n161 = Concatenate Strings("FAIL *" ("f"), w438) -> (w437:string)
              n162 = Select(t="PASS", s=w417, f=w423) -> (s? t:f=w390:string)
              n163 = Select(t="PASS", s=w412, f=w426) -> (s? t:f=w394:string)
              n164 = Select(t="PASS", s=w411, f=w429) -> (s? t:f=w393:string)
              n165 = Select(t="PASS", s=w434, f=w432) -> (s? t:f=w392:string)
              n166 = Select(t="PASS", s=w435, f=w437) -> (s? t:f=w391:string)
              n167 = local write "TX_DC"(w390) -> ()
              n168 = local write "TX_POW"(w394) -> ()
              n169 = local write "TX_S11"(w393) -> ()
              n170 = local write "TX_H2"(w392) -> ()
              n171 = local write "TX_FLAT"(w391) -> ()
            }
            frame #6 {
              n172 = local read "TX_FLAT"() -> (w443:string)
              n173 = local read "Tx_Header"() -> (w457:string[])
              n174 = local read "Tx_Header_data"() -> (w458:string[])
              n175 = local read "TX_DC"() -> (w451:string)
              n176 = local read "TX_H2"() -> (w445:string)
              n177 = local read "TX_POW"() -> (w449:string)
              n178 = local read "TX_S11"() -> (w446:string)
              n179 = Array Size(array=w457) -> (size(s)=w456:i32)
              n180 = Insert Into Array(array=w457, index=w456, new element #1="%TX_DC" ("new element/subarray"), new element #2="%TX_POW" ("new element/subarray"), new element #3="%TX_S11" ("new element/subarray"), new element #4="%TX_H2" ("new element/subarray"), new element #5="%TX_FLAT" ("new element/subarray")) -> (w454:string[])
              n181 = Insert Into Array(array=w458, index=w456, new element #1=w451, new element #2=w449, new element #3=w446, new element #4=w445, new element #5=w443) -> (w455:string[])
              n182 = Build Array(w454, w455) -> (w453:string[][])
              n183 = Transpose 2D Array(2D array=w453) -> (transposed array=w442:string[][])
            }
          }
        }
      }
      n184 = case shown="True" w92 {
        tunnel: w93 -> [_ w197]
        tunnel: [string[][] [] w196] -> w87
        tunnel: w89 -> [w193 w195]
        tunnel: [w193 w195] -> w88
        frame False {
        }
        frame True {
          n185 = flat-sequence {
            tunnel: [w201] -> w198
            tunnel: w197 -> [w201]
            tunnel: w198 -> [w207]
            tunnel: [w235] -> w200
            tunnel: w200 -> [w258]
            tunnel: [w256] -> w199
            tunnel: w199 -> [w269]
            tunnel: [w300] -> w196
            frame #0 {
              w203 = string[][] [] ("TX_DAT")
              w204 = string[] [] ("TxAtt_Header_data")
              w202 = ""
              "Rx_Header" <- w204
              "Rx_Header_data" <- w204
              "Rx_Test Name" <- w202
              "RX_DC" <- w202
              "RX_G" <- w202
              "RX_NF" <- w202
              "RX_DAT" <- w203
              "Rx_DataLength" <- 0 ("Tx_DataLength")
              "Rx_Result" <- i32[][] [] ("Tx_Result")
              "Rx_Data" <- w203
              "RX_ResultFile" <- w202
            }
            frame #1 {
              # "Get The file"
              n186 = Path To String(path=w207) -> (string=w208:string)
              n187 = call-poly <vilib>:"Read Delimited Spreadsheet.vi"("file path (dialog if empty)"=w207, "delimiter (\\t)"="," ("delimiter (\\t)")) -> ("all rows"=w209:string[][])  [unwired: 8 in, 5 out]
              n188 = local write "RX_ResultFile"(w208) -> ()
              n189 = local write "Rx_Data"(w209) -> ()
            }
            frame #2 {
              # "Create The Header"
              n190 = local read "Rx_Data"() -> (w217:string[][])
              n191 = Build Array("#Test Name:" ("regular expression"), "#MSN:" ("regular expression"), "#ESN:" ("regular expression"), "#TestOperator:" ("regular expression"), "#Test_Bench_Name:" ("regular expression"), "#Test Parameters File Name:" ("regular expression"), "#Gitlog Commit:" ("regular expression"), "#LotID:" ("regular expression"), "#SW_Version: " ("regular expression"), "#Result File Path:" ("regular expression")) -> (w215:string[])
              n192 = Index Array(array=w217, index (col)=0 ("disabled index (col)")) -> (element=w225:string[])  [unwired: 1 in]
              n193 = for {
                tunnel: w215 -> [w228] mode=indexing
                tunnel: w225 -> [w227]
                tunnel: [w226] -> w216 mode=indexing
                n194 = for {
                  tunnel: w228 -> [w229]
                  tunnel: [w231] -> w226
                  tunnel: w227 -> [w230] mode=indexing
                  stop <- w234 stop-if-true
                  n195 = Match Pattern(string=w230, regular expression=w229) -> (match substring=w233:string, after substring=w232:string)  [unwired: 1 in, 2 out]
                  n196 = Equal?(x=w233, y=w229) -> (x = y?=w234:bool)
                  n197 = call <vilib>:"Trim Whitespace.vi"("string"=w232) -> ("trimmed string"=w231:string)  [unwired: 1 in]
                }
              }
              n198 = local write "Rx_Header"(w215) -> ()
              n199 = local write "Rx_Header_data"(w216) -> ()
            }
            frame #3 {
              # "Find The Data Section"
              n200 = local read "Rx_Data"() -> (w244:string[][])
              n201 = Index Array(array=w244, index (col)=0 ("disabled index (col)")) -> (element=w237:string[])  [unwired: 1 in]
              n202 = for {
                tunnel: w237 -> [w254] mode=indexing
                tunnel: [w250] -> w238
                i -> [w250]
                stop <- w251 stop-if-true
                w252 = "#Begin Data" ("regular expression")
                n203 = Match Pattern(string=w254, regular expression=w252) -> (match substring=w253:string)  [unwired: 1 in, 3 out]
                n204 = Equal?(x=w253, y=w252) -> (x = y?=w251:bool)
              }
              n205 = Increment(x=w238) -> (x+1=w240:i32)
              n206 = Increment(x=w240) -> (x+1=w243:i32)
              "Rx_DataHeaderRow" <- w243
              n207 = Index Array(array=w244, index (row)=w240) -> (element=w239:string[])  [unwired: 1 in]
              n208 = for {
                tunnel: w239 -> [w249] mode=indexing
                tunnel: [w245] -> w241
                i -> [w245]
                stop <- w246 stop-if-true
                w247 = "pass/fail(Bool)" ("regular expression")
                n209 = Match Pattern(string=w249, regular expression=w247) -> (match substring=w248:string)  [unwired: 1 in, 3 out]
                n210 = Equal?(x=w248, y=w247) -> (x = y?=w246:bool)
              }
              n211 = Decrement(x=w241) -> (x-1=w242:i32)
              n212 = Array Subset(array=w244, index (row)=w243, index (col)=w242) -> (w235:string[][])  [unwired: 2 in]
            }
            frame #4 {
              # "Get the P/F result, parse the charactors"
              n213 = Index Array(array=w258, index (col)=0 ("disabled index (col)")) -> (element=w259:string[])  [unwired: 1 in]
              n214 = for {
                tunnel: w259 -> [w266] mode=indexing
                tunnel: [w263] -> w256 mode=indexing
                tunnel: [w260] -> w255
                i -> [w261]
                n215 = Increment(x=w261) -> (x+1=w260:i32)
                n216 = Scan From String(format string="%1b%1b%1b", input string=w266) -> (output 1=w262:i32, output 2=w265:i32, output 3=w264:i32)  [unwired: 5 in, 3 out]
                n217 = Build Array(w262, w265, w264) -> (w263:i32[])
              }
              n218 = local write "Rx_DataLength"(w255) -> ()
              n219 = local write "Rx_Result"(w256) -> ()
            }
            frame #5 {
              n220 = Index Array(array=w269, index (col) #1=0 ("disabled index (col)")) -> (element #1=w287:i32[], element #2=w286:i32[], element #3=w285:i32[])  [unwired: 5 in]
              n221 = local read "Rx_DataLength"() -> (w282:i32)
              n222 = local read "Rx_DataLength"() -> (w281:i32)
              n223 = local read "Rx_DataLength"() -> (w276:i32)
              n224 = Add Array Elements(numeric array=w287) -> (sum=w283:i32)
              n225 = Add Array Elements(numeric array=w286) -> (sum=w280:i32)
              n226 = Add Array Elements(numeric array=w285) -> (sum=w277:i32)
              n227 = Subtract(x=w282, y=w283) -> (x-y=w288:i32)
              n228 = Subtract(x=w281, y=w280) -> (x-y=w291:i32)
              n229 = Subtract(x=w276, y=w277) -> (x-y=w294:i32)
              n230 = Equal?(x=w282, y=w283) -> (x = y?=w284:bool)
              n231 = Equal?(x=w281, y=w280) -> (x = y?=w279:bool)
              n232 = Equal?(x=w276, y=w277) -> (x = y?=w278:bool)
              n233 = Number To Decimal String(number=w288) -> (decimal integer string=w290:string)  [unwired: 1 in]
              n234 = Number To Decimal String(number=w291) -> (decimal integer string=w293:string)  [unwired: 1 in]
              n235 = Number To Decimal String(number=w294) -> (decimal integer string=w296:string)  [unwired: 1 in]
              n236 = Concatenate Strings("FAIL *" ("f"), w290) -> (w289:string)
              n237 = Concatenate Strings("FAIL *" ("f"), w293) -> (w292:string)
              n238 = Concatenate Strings("FAIL *" ("f"), w296) -> (w295:string)
              n239 = Select(t="PASS", s=w284, f=w289) -> (s? t:f=w297:string)
              n240 = Select(t="PASS", s=w279, f=w292) -> (s? t:f=w298:string)
              n241 = Select(t="PASS", s=w278, f=w295) -> (s? t:f=w299:string)
              n242 = local write "RX_DC"(w297) -> ()
              n243 = local write "RX_NF"(w299) -> ()
              n244 = local write "RX_G"(w298) -> ()
            }
            frame #6 {
              n245 = local read "Rx_Header"() -> (w311:string[])
              n246 = local read "Rx_Header_data"() -> (w312:string[])
              n247 = local read "RX_DC"() -> (w305:string)
              n248 = local read "RX_NF"() -> (w301:string)
              n249 = local read "RX_G"() -> (w303:string)
              n250 = Array Size(array=w311) -> (size(s)=w310:i32)
              n251 = Insert Into Array(array=w311, index=w310, new element #1="%RX_DC" ("new element/subarray"), new element #2="%RX_GAIN" ("new element/subarray"), new element #3="%RX_NF" ("new element/subarray")) -> (w308:string[])
              n252 = Insert Into Array(array=w312, index=w310, new element #1=w305, new element #2=w303, new element #3=w301) -> (w309:string[])
              n253 = Build Array(w308, w309) -> (w307:string[][])
              n254 = Transpose 2D Array(2D array=w307) -> (transposed array=w300:string[][])
            }
          }
        }
      }
      n255 = local write "RX_DAT"(w87) -> ()
      n256 = local write "TX-ATT_DAT"(w85) -> ()
      n257 = local write "TX_DAT"(w86) -> ()
    }
    frame #3 {
      n258 = local read "RunATTEN(t)"() -> (w459:bool)
      n259 = case shown="True" w459 {
        tunnel: w461 -> [w462 w481]
        tunnel: [w462 w476] -> w460
        frame False {
        }
        frame True {
          n260 = local read "RunATTEN(t)"() -> (w486:bool)
          n261 = local read "reportfile"() -> (w468:path)
          n262 = local read "RunTx(t)"() -> (w487:bool)
          n263 = local read "RunRx(t)"() -> (w485:bool)
          n264 = Path To String(path=w468) -> (string=w467:string)
          n265 = Or(x=w486, y=w487) -> (x .or. y?=w488:bool)
          n266 = Build Array("#Report File: " ("element"), w467) -> (w466:string[])
          n267 = local read "TX-ATT_DAT"() -> (w494:string[][])
          n268 = local read "TX_DAT"() -> (w496:string[][])
          n269 = local read "RX_DAT"() -> (w497:string[][])
          n270 = local read "reportfile"() -> (w495:path)
          n271 = local read "reportfile"() -> (w489:path)
          n272 = local read "reportfile"() -> (w490:path)
          n273 = Insert Into Array(array=w494, new element=string[] [] ("new element/subarray")) -> (w491:string[][])  [unwired: 2 in]
          n274 = Insert Into Array(array=w496, new element=string[] [] ("new element/subarray")) -> (w492:string[][])  [unwired: 2 in]
          n275 = Insert Into Array(array=w497, new element=string[] [] ("new element/subarray")) -> (w493:string[][])  [unwired: 2 in]
          n276 = case shown="True" w486 {
            tunnel: w495 -> [_ w520]
            tunnel: w491 -> [_ w518]
            tunnel: w481 -> [w515 w517]
            tunnel: [w515 w516] -> w480
            frame False {
            }
            frame True {
              n277 = call-poly <vilib>:"Write Delimited Spreadsheet.vi"("file path (dialog if empty)"=w520, "2D data"=w518, "append to file? (new file:F)"=FALSE, "error in (no error)"=w517, "delimiter (\\t)"="," ("delimiter (\\t)")) -> ("error out"=w516:errorcluster)  [unwired: 9 in, 1 out]
            }
          }
          n278 = case shown="True" w487 {
            tunnel: w486 -> [_ w512]
            tunnel: w489 -> [_ w513]
            tunnel: w492 -> [_ w511]
            tunnel: w480 -> [w508 w510]
            tunnel: [w508 w509] -> w479
            frame False {
            }
            frame True {
              n279 = call-poly <vilib>:"Write Delimited Spreadsheet.vi"("file path (dialog if empty)"=w513, "2D data"=w511, "append to file? (new file:F)"=w512, "error in (no error)"=w510, "delimiter (\\t)"="," ("delimiter (\\t)")) -> ("error out"=w509:errorcluster)  [unwired: 9 in, 1 out]
            }
          }
          n280 = case shown="True" w485 {
            tunnel: w488 -> [_ w505]
            tunnel: w490 -> [_ w506]
            tunnel: w493 -> [_ w504]
            tunnel: w479 -> [w501 w503]
            tunnel: [w501 w502] -> w477
            frame False {
            }
            frame True {
              n281 = call-poly <vilib>:"Write Delimited Spreadsheet.vi"("file path (dialog if empty)"=w506, "2D data"=w504, "append to file? (new file:F)"=w505, "error in (no error)"=w503, "delimiter (\\t)"="," ("delimiter (\\t)")) -> ("error out"=w502:errorcluster)  [unwired: 9 in, 1 out]
            }
          }
          n282 = call-poly <vilib>:"Read Delimited Spreadsheet.vi"("file path (dialog if empty)"=w468, "error in (no error)"=w477, "delimiter (\\t)"="," ("delimiter (\\t)")) -> ("new file path (Not A Path if cancelled)"=w464:path, "all rows"=w471:string[][], "error out"=w476:errorcluster)  [unwired: 7 in, 3 out]
          n283 = Insert Into Array(array=w471, index (row)=0, new element=w466) -> (w469:string[][])  [unwired: 1 in]
          n284 = for {
            tunnel: [w499] -> w475 mode=indexing
            tunnel: w469 -> [w498] mode=indexing
            n285 = Array To Spreadsheet String(array=w498, 3:"%s" ("format string")) -> (spreadsheet string=w499:string)  [unwired: 1 in]
          }
          n286 = Path To String(path=w464) -> (string=→"reportfile(str)":string)
          n287 = Array To Spreadsheet String(delimiter (Tab)="", array=w475, 3:"" ("format string")) -> (spreadsheet string=w472:string)
          n288 = Two Button Dialog(message=w472) -> ()  [unwired: 2 in, 1 out]
        }
      }
    }
  }
  "error out" <- w10
